vi "message_popup.vi"(7 "Warning(T)/Info(F)":bool, 8 "error_in":errorcluster, 9 "Message":string, 10 "Title":string, 11 "Button Label":string) -> (0 "error_out":errorcluster)   [LabVIEW 2020]
uses:
  AULocalize/SubVIs/Get Localized Phrase Compact Interface 0D.vi
panel:
  out "Project Title 2":string
  out "Message copy":string
  in  "OK":bool
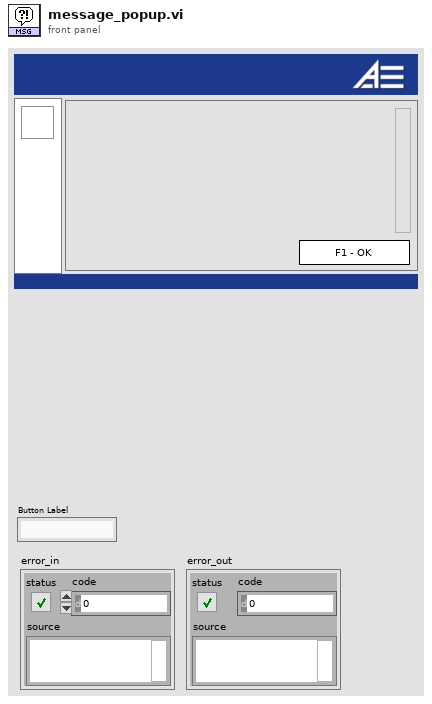
[diagram p1: front panel]
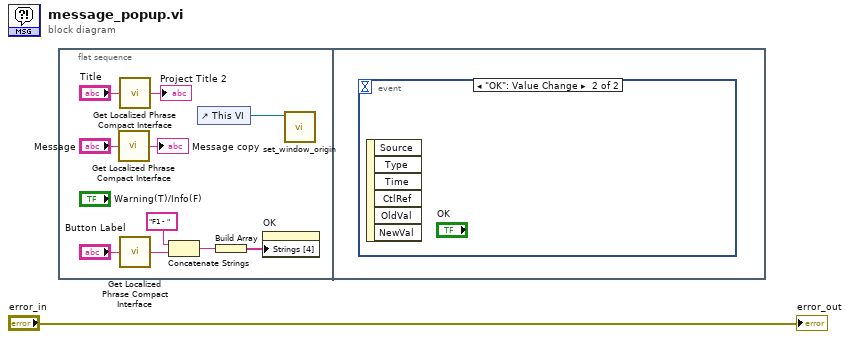
[diagram p0: block diagram]
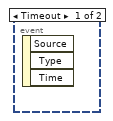
[diagram p2: hidden frame]
diagram:
  n1 = flat-sequence {
    frame #0 {
      n2 = call-poly "Get Localized Phrase Compact Interface.vi"("Key"="Message") -> ("Translated Phrase"=→"Message copy":string)
      n3 = call-poly "Get Localized Phrase Compact Interface.vi"("Key"="Title") -> ("Translated Phrase"=→"Project Title 2":string)
      n4 = call-poly "Get Localized Phrase Compact Interface.vi"("Key"="Button Label") -> ("Translated Phrase"=w2:string)
      n5 = Concatenate Strings("F1 - ", w2) -> (w6:string)
      n6 = control-ref of="This VI"() -> (w5:refnum<vi>)
      n7 = Build Array(w6) -> (w11:string[])
      n8 = property on="OK" class="Bool"("Strings [4]"=w11) -> ()  [unwired: 2 in, 2 out]
      n9 = call "set_window_origin.vi"("this_vi_reference"=w5) -> ()  [unwired: 10 in, 1 out]
    }
    frame #1 {
      n10 = event shown="[1] \"OK\": Value Change" {
        selector: _ -> [_ _]
        dyn-events: _ -> [_ _]
        timeout: _ -> [_ _]
        event Timeout {
          n11 = event-data() -> ()  [unwired: 1 in, 3 out]
        }
        event "OK": Value Change {
          n12 = event-data() -> ()  [unwired: 1 in, 6 out]
        }
      }
    }
  }
  "error_out" <- "error_in"
